vi "Cunningham Correction Factor.vi"(1 "T (K)":dbl, 2 "P (mb)":dbl, 3 "D (mm)":dbl) -> (0 "Cc":dbl)   [LabVIEW 2015]
doc: "Calculate the Cuningham correction factor. The methodology uses that outlined in Hinds [1999] - for particles larger than 100 nm, use equation 3.19; for those smaller, use the estimate in 3.20."
uses:
  Atmospheric/Atmospheric Library.lvlib
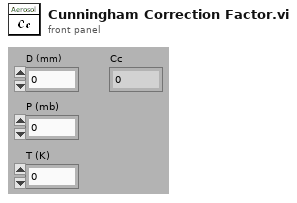
[diagram p1: front panel]
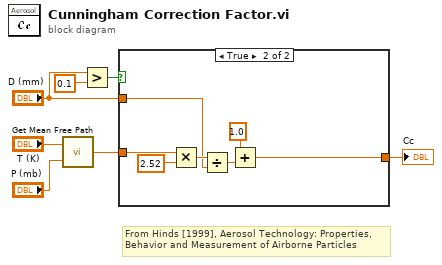
[diagram p0: block diagram]
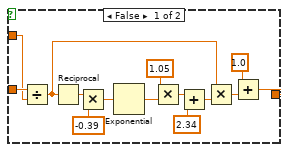
[diagram p2: hidden frame]
diagram:
  # "From Hinds [1999], Aerosol Technology: Properties, Behavior and Measurement of Airborne Particles"
  n1 = call "Get Mean Free Path.vi"("P"="P (mb)", "T"="T (K)") -> ("l (mm)"=w3:dbl)
  n2 = Greater?(x="D (mm)", y=0.1) -> (0:w6:bool)
  n3 = case shown="True" w6 {
    tunnel: w3 -> [w20 w27]
    tunnel: "D (mm)" -> [w19 w24]
    tunnel: [w10 w22] -> w1
    frame False {
      n4 = Divide(x=w20, y=w19) -> (x/y=w8:dbl)
      n5 = Reciprocal(x=w8) -> (1/x=w15:dbl)
      n6 = Multiply(x=w15, y=-0.39) -> (x*y=w14:dbl)
      n7 = Exponential(1:w14) -> (0:w13:dbl)
      n8 = Multiply(x=1.05, y=w13) -> (x*y=w12:dbl)
      n9 = Add(x=w12, y=2.34) -> (x+y=w9:dbl)
      n10 = Multiply(x=w8, y=w9) -> (x*y=w11:dbl)
      n11 = Add(x=1.0, y=w11) -> (x+y=w10:dbl)
    }
    frame True {
      n12 = Multiply(x=w27, y=2.52) -> (x*y=w25:dbl)
      n13 = Divide(x=w25, y=w24) -> (x/y=w23:dbl)
      n14 = Add(x=1.0, y=w23) -> (x+y=w22:dbl)
    }
  }
  "Cc" <- w1
